vi "CameraOverlayImageGFV.vi"(8 "error in (no error)":errorcluster, 10 "Enum":T1=enum."Get Image overlay", 11 "Data in":variant) -> (0 "error out":errorcluster, 3 "Data Out":variant)   [LabVIEW 2017]
doc: "Image overlay of the camera is saved temp to fix the problem that the overlay is destroyed once a new image is acquired."
uses:
  CameraImageOverlayEnum.ctl
  <vilib>/vision/Image Controls.llb/IMAQ Image.ctl
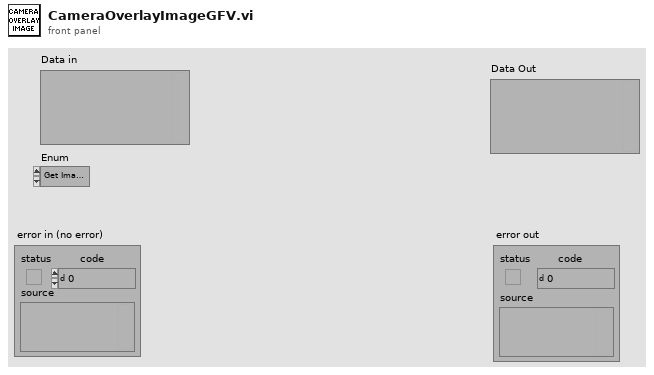
[diagram p1: front panel]
types:
  T1 = typedef "CameraImageOverlayEnum.ctl" = enum16{"Shutdown", "Get Image overlay", "Save image overlay", "Init"}
  T2 = typedef "IMAQ Image.ctl" = refnum<image>
  T3 = typedef "Image Type" = u32
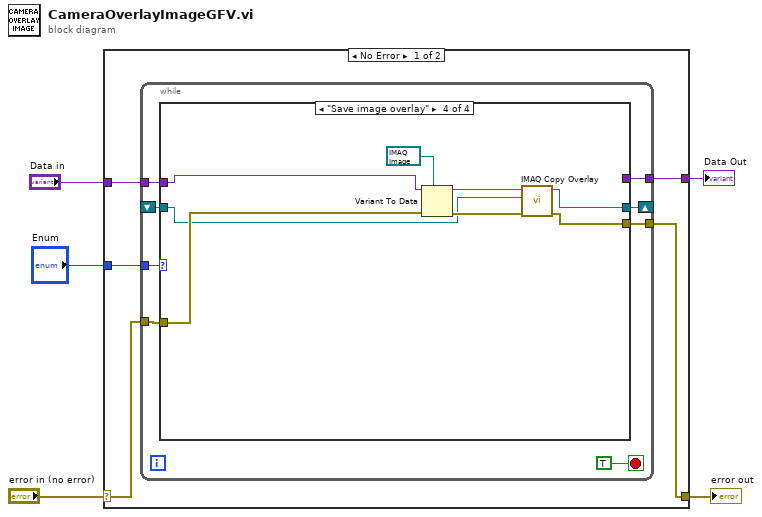
[diagram p0: block diagram]
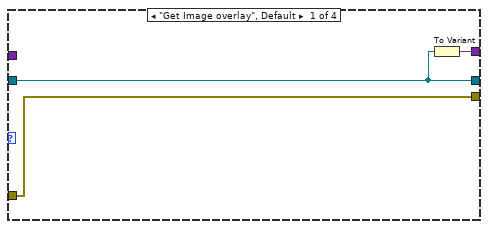
[diagram p2: hidden frame]
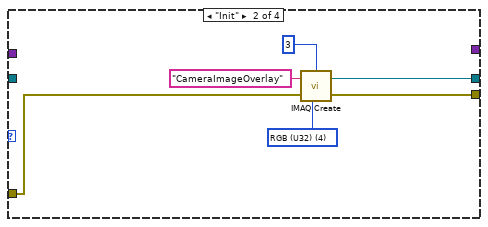
[diagram p3: hidden frame]
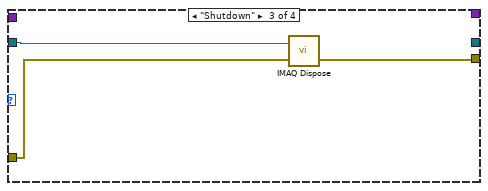
[diagram p4: hidden frame]
diagram:
  n1 = case shown="No Error" "error in (no error)" {
    selector: "error in (no error)" -> [w9 w39]
    tunnel: [w8 w39] -> w4
    tunnel: "Enum" -> [w10 _]
    tunnel: "Data in" -> [w7 _]
    tunnel: [w6 _] -> w1
    frame No Error {
      n2 = while {
        tunnel: w10 -> [w17]
        tunnel: w9 -> [w16]
        tunnel: [w15] -> w8
        shift-right: [w14] -> _
        shift-left: _ -> [w13]
        tunnel: w7 -> [w12]
        tunnel: [w11] -> w6
        stop <- TRUE stop-if-true
        n3 = case shown="\"Save image overlay\"" w17 {
          tunnel: w16 -> [w21 w25 w29 w32]
          tunnel: [w21 w24 w28 w33] -> w15
          tunnel: [w20 w23 _ w34] -> w14
          tunnel: w13 -> [w20 _ w30 w31]
          tunnel: w12 -> [_ _ _ w38]
          tunnel: [w19 _ _ _] -> w11
          frame "Get Image overlay", Default {
            n4 = To Variant(anything=w20) -> (Variant=w19:variant)
          }
          frame "Init" {
            w26 = T3 4 items=["Grayscale (U8)", "Grayscale (I16)", "Grayscale (SGL)", "Complex (CSG)", "RGB (U32)", "HSL (U32)", "RGB (U64)", "Grayscale (U16)"] ("Image Type")
            n5 = call "IMAQ Create"("Border Size"=3, "Image Name"="CameraImageOverlay", "Image Type"=w26, "error in (no error)"=w25) -> ("New Image"=w23:T2, "error out"=w24:errorcluster)  [unwired: 1 in]
          }
          frame "Shutdown" {
            n6 = call "IMAQ Dispose"("Image"=w30, "error in (no error)"=w29) -> ("error out"=w28:errorcluster)  [unwired: 4 in]
          }
          frame "Save image overlay" {
            n7 = Variant To Data(error in=w32, type=T2 refnum ("New Image"), Variant=w38) -> (data=w35:T2, error out=w36:errorcluster)
            n8 = call "IMAQ Copy Overlay"("error in (no error)"=w36, "Image Dst"=w31, "Image Src"=w35) -> ("error out"=w33:errorcluster, "Image Dst Out"=w34:T2)  [unwired: 7 in]
          }
        }
      }
    }
    frame Error {
    }
  }
  "error out" <- w4
  "Data Out" <- w1
